vi "Stepper.vi"(8 "error in (no error)":errorcluster, 11 "VISA Refnum in":refnum<visa-resource-name>) -> (0 "error out":errorcluster, 3 "VISA Refnum out":refnum<visa-resource-name>)   [LabVIEW 2016]
panel:
  in  "stop":bool
  in  "Down Button":bool
  in  "UP\n Button":bool
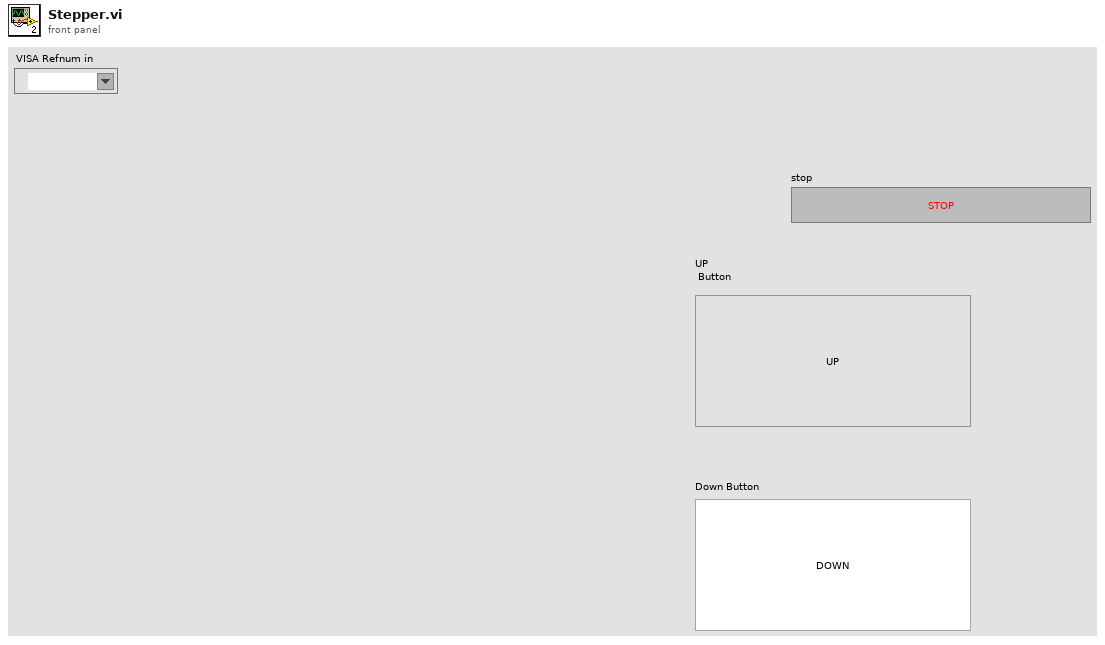
[diagram p1: front panel]
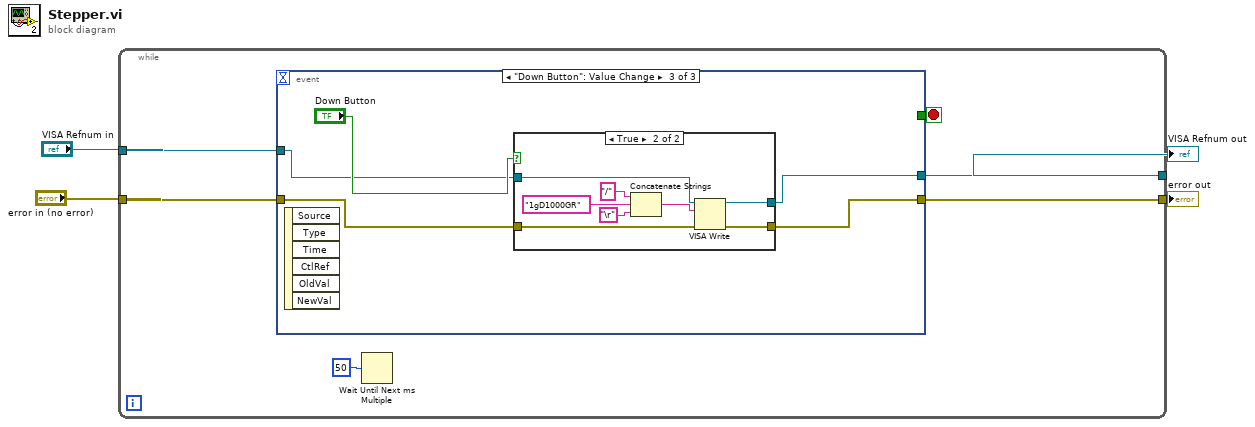
[diagram p0: block diagram]
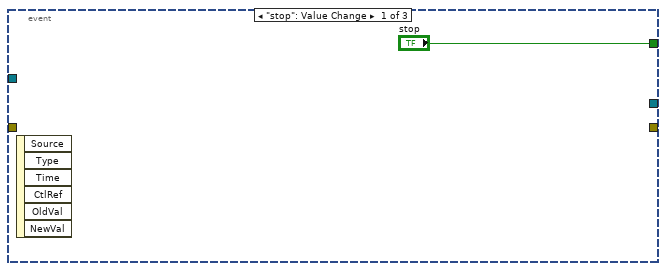
[diagram p2: hidden frame]
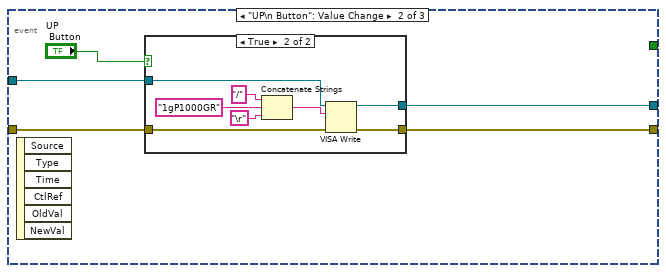
[diagram p3: hidden frame]
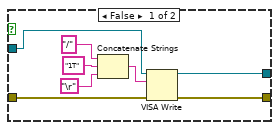
[diagram p4: hidden frame]
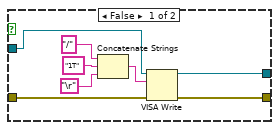
[diagram p5: hidden frame]
diagram:
  n1 = while {
    tunnel: "VISA Refnum in" -> [w7]
    tunnel: [w9] -> w3
    tunnel: "error in (no error)" -> [w6]
    tunnel: [w8] -> w4
    stop <- w10 stop-if-true
    n2 = event shown="[2] \"Down Button\": Value Change" {
      selector: _ -> [_ _ _]
      dyn-events: _ -> [_ _ _]
      timeout: _ -> [_ _ _]
      tunnel: ["stop" _ _] -> w10
      tunnel: [_ w14 w34] -> w9
      tunnel: [_ w13 w33] -> w8
      tunnel: w7 -> [_ w16 w36]
      tunnel: w6 -> [_ w15 w35]
      event "stop": Value Change {
        n3 = event-data() -> ()  [unwired: 1 in, 6 out]
      }
      event "UP\n Button": Value Change {
        n4 = event-data() -> ()  [unwired: 1 in, 6 out]
        n5 = case shown="True" "UP\n Button" {
          tunnel: w16 -> [w20 w32]
          tunnel: w15 -> [w19 w31]
          tunnel: [w18 w26] -> w14
          tunnel: [w17 w25] -> w13
          frame False {
            n6 = Concatenate Strings("/" ("string to write 2"), "1T" ("string"), "\r") -> (w23:string)
            n7 = VISA Write(VISA resource name=w20, write buffer=w23, error in (no error)=w19) -> (VISA resource name out=w18:refnum<visa-resource-name>, error out=w17:errorcluster)  [unwired: 1 out]
          }
          frame True {
            n8 = Concatenate Strings("/" ("string to write 2"), "1gP1000GR" ("string"), "\r") -> (w29:string)
            n9 = VISA Write(VISA resource name=w32, write buffer=w29, error in (no error)=w31) -> (VISA resource name out=w26:refnum<visa-resource-name>, error out=w25:errorcluster)  [unwired: 1 out]
          }
        }
      }
      event "Down Button": Value Change {
        n10 = event-data() -> ()  [unwired: 1 in, 6 out]
        n11 = case shown="True" "Down Button" {
          tunnel: w36 -> [w41 w53]
          tunnel: w35 -> [w40 w52]
          tunnel: [w39 w47] -> w34
          tunnel: [w38 w46] -> w33
          frame False {
            n12 = Concatenate Strings("/" ("string to write 2"), "1T" ("string"), "\r") -> (w44:string)
            n13 = VISA Write(VISA resource name=w41, write buffer=w44, error in (no error)=w40) -> (VISA resource name out=w39:refnum<visa-resource-name>, error out=w38:errorcluster)  [unwired: 1 out]
          }
          frame True {
            n14 = Concatenate Strings("/" ("string to write 2"), "1gD1000GR" ("string"), "\r") -> (w50:string)
            n15 = VISA Write(VISA resource name=w53, write buffer=w50, error in (no error)=w52) -> (VISA resource name out=w47:refnum<visa-resource-name>, error out=w46:errorcluster)  [unwired: 1 out]
          }
        }
      }
    }
    n16 = Wait Until Next ms Multiple(millisecond multiple=u32 50) -> ()  [unwired: 1 out]
  }
  "error out" <- w4
  "VISA Refnum out" <- w3
